vi "DSK.vi"() -> (0 "Total Money":i32, 1 "All TRansactions":string[][](table), 2 "Array 3":string[](array[string]), 3 "Current Transaction":string[][](table))   [LabVIEW 2023]
uses:
  <vilib>/Utility/file.llb/Read Delimited Spreadsheet (string).vi
panel:
  out "Waveform Chart":dbl(graph)
  in  "?":bool
  out "x .and. y?":bool
  out "Array 4":string[][](array[string])
  out "Array":string[][](array[string])
  out "Current Rows num":i32
  out "All Rows num":i32
  out "Array 2":string[](array[string])
  out "Transaction":string
  in  "Transaction Type":T1(ring)
  in  "file path":path
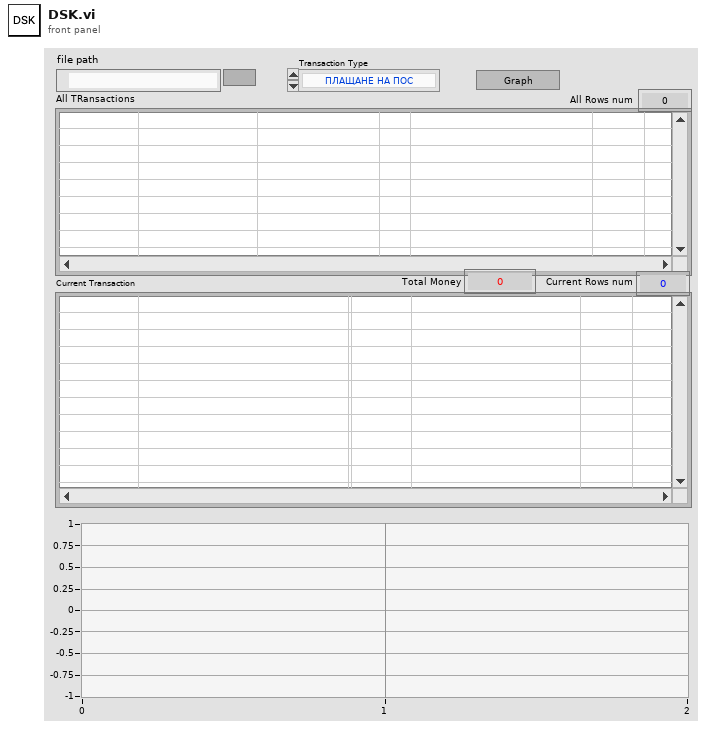
[diagram p1: front panel]
types:
  T1 = enum16{"ПЛАЩАНЕ НА ПОС", "СБКО", "ТЕГЛЕНЕ", "ЗАЕМ", "BREZOVO", "VIVACOM", "ЕЛЕКТРОХОЛД", "ЕВН", "ЗАПЛАТА", "АВАНС", "НЕТ", "ТРАНСФЕР"}
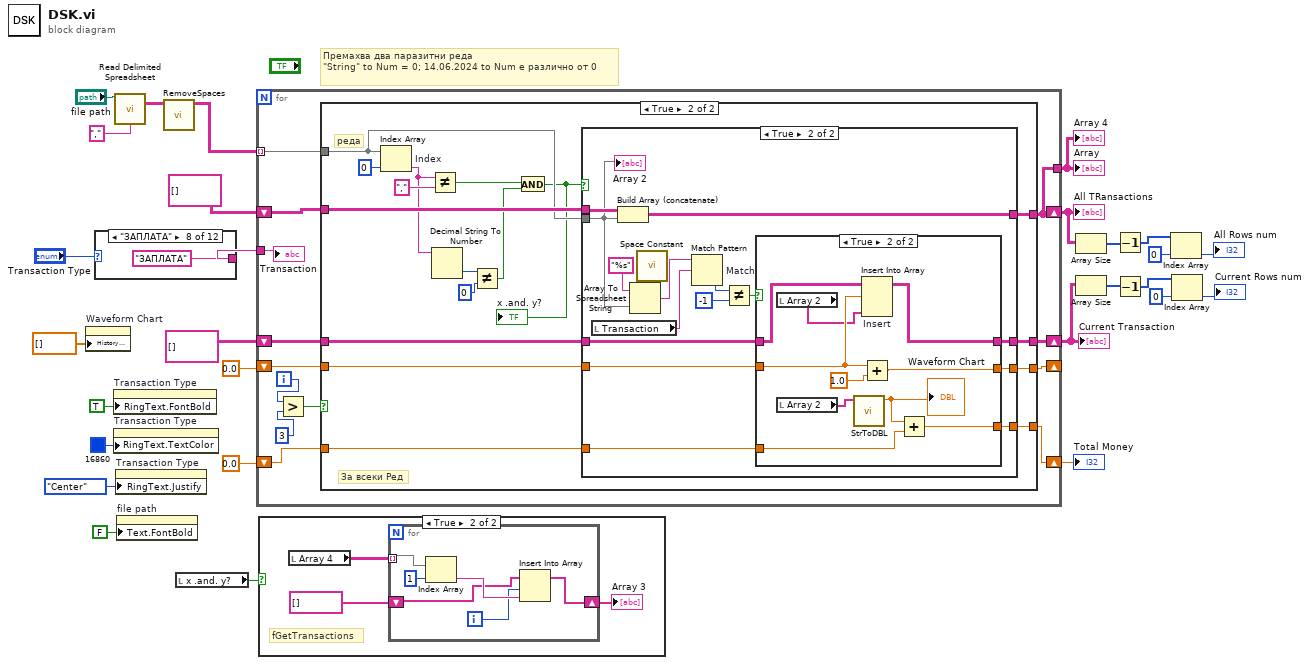
[diagram p0: block diagram]
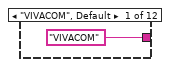
[diagram p3: hidden frame]
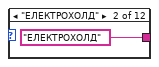
[diagram p4: hidden frame]
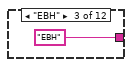
[diagram p5: hidden frame]
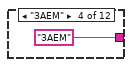
[diagram p6: hidden frame]
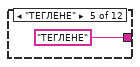
[diagram p7: hidden frame]
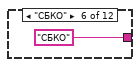
[diagram p8: hidden frame]
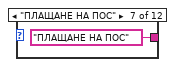
[diagram p9: hidden frame]
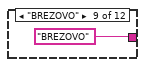
[diagram p10: hidden frame]
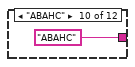
[diagram p11: hidden frame]
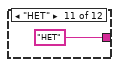
[diagram p12: hidden frame]
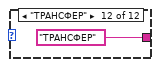
[diagram p13: hidden frame]
diagram:
  # "Премахва два паразитни реда\n\"String\" to Num = 0; 14.06.2024 to Num е различно от 0"
  n1 = property on="Waveform Chart" class="WFChart (strict)"("History Data"=dbl[] []) -> ()  [unwired: 2 in, 2 out]
  n2 = case shown="\"ЗАПЛАТА\"" "Transaction Type" {
    tunnel: ["VIVACOM" "ЕЛЕКТРОХОЛД" "ЕВН" "ЗАЕМ" "ТЕГЛЕНЕ" "СБКО" "ПЛАЩАНЕ НА ПОС" "ЗАПЛАТА" "BREZOVO" "АВАНС" "НЕТ" "ТРАНСФЕР"] -> w27
    frame "VIVACOM", Default {
    }
    frame "ЕЛЕКТРОХОЛД" {
    }
    frame "ЕВН" {
    }
    frame "ЗАЕМ" {
    }
    frame "ТЕГЛЕНЕ" {
    }
    frame "СБКО" {
    }
    frame "ПЛАЩАНЕ НА ПОС" {
    }
    frame "ЗАПЛАТА" {
    }
    frame "BREZOVO" {
    }
    frame "АВАНС" {
    }
    frame "НЕТ" {
    }
    frame "ТРАНСФЕР" {
    }
  }
  n3 = property on="Transaction Type" class="Enum (strict)"("RingText.FontBold"=TRUE ("Ring Text.Font:Bold")) -> ()  [unwired: 2 in, 2 out]
  n4 = property on="Transaction Type" class="Enum (strict)"("RingText.TextColor"=u32 16860 ("Ring Text.Text Colors:Text Color")) -> ()  [unwired: 2 in, 2 out]
  n5 = call-poly <vilib>:"Read Delimited Spreadsheet.vi"("file path (dialog if empty)"="file path", "delimiter (\\t)"="," ("delimiter (\\t)")) -> ("all rows"=w2:string[][])  [unwired: 8 in, 5 out]
  n6 = property on="Transaction Type" class="Enum (strict)"("RingText.Justify"=enum16{"Left", "Center", "Right"}."Center" ("Ring Text.Justification")) -> ()  [unwired: 2 in, 2 out]
  n7 = property on="file path" class="Path"("Text.FontBold"=FALSE ("Path Text.Font:Bold")) -> ()  [unwired: 2 in, 2 out]
  n8 = call "RemoveSpaces.vi"("all rows"=w2) -> ("Array 2"=w3:string[][])  [unwired: 10 in]
  n9 = local read "x .and. y?"() -> (w4:bool)
  n10 = for {
    tunnel: w27 -> [w49]
    tunnel: w3 -> [w45] mode=indexing
    shift-right: [w41] -> w19
    shift-left: string[][] [] -> [w50]
    shift-right: [w44] -> w6
    shift-left: string[][] [] -> [w48]
    shift-right: [w47] -> _
    shift-left: 0.0 ("y") -> [w46]
    shift-right: [w43] -> w18
    shift-left: 0.0 ("y") -> [w42]
    tunnel: [w41] -> w7
    i -> [w53]
    n11 = Greater?(x=w53, y=3) -> (0:w51:bool)
    n12 = case shown="True" w51 {
      tunnel: w45 -> [_ w65]
      tunnel: [w57 w72] -> w41
      tunnel: w50 -> [w57 w71]
      tunnel: [w56 w64] -> w44
      tunnel: w48 -> [w56 w63]
      tunnel: [w55 w62] -> w47
      tunnel: w46 -> [w55 w61]
      tunnel: [w54 w60] -> w43
      tunnel: w42 -> [w54 w59]
      frame False {
      }
      frame True {
        # "реда"
        # "За всеки Ред"
        n13 = Index Array "Index"(array=w65, index=0) -> (element=w70:string)
        n14 = Not Equal?(x=w70, y=",") -> (x != y?=w67:bool)
        n15 = Decimal String To Number(string=w70) -> (number=w69:i32)  [unwired: 2 in, 1 out]
        n16 = Not Equal?(x=w69, y=0) -> (x != y?=w66:bool)
        n17 = And(x=w67, y=w66) -> (x .and. y?=w58:bool)
        "x .and. y?" <- w58
        n18 = case shown="True" w58 {
          tunnel: w65 -> [_ w79]
          tunnel: [w78 w80] -> w72
          tunnel: w71 -> [w78 w94]
          tunnel: [w77 w83] -> w64
          tunnel: w63 -> [w77 w86]
          tunnel: [w76 w85] -> w62
          tunnel: w61 -> [w76 w84]
          tunnel: [w75 w82] -> w60
          tunnel: w59 -> [w75 w81]
          frame False {
          }
          frame True {
            n19 = local read "Transaction"() -> (w90:string)
            n20 = Build Array (concatenate)(w94, w79) -> (w80:string[][])
            n21 = call <vilib>:"Space Constant.vi"() -> ("String"=w92:string)
            n22 = Array To Spreadsheet String(delimiter (Tab)=w92, array=w79, 3:"%s" ("format string")) -> (spreadsheet string=w91:string)
            n23 = Match Pattern "Match"(string=w91, regular expression=w90) -> (offset past match=w89:i32)  [unwired: 1 in, 3 out]
            n24 = Not Equal?(x=w89, y=-1) -> (x != y?=w87:bool)
            n25 = case shown="True" w87 {
              tunnel: [w97 w99] -> w83
              tunnel: w86 -> [w97 w107]
              tunnel: [w96 w105] -> w85
              tunnel: w84 -> [w96 w104]
              tunnel: [w95 w101] -> w82
              tunnel: w81 -> [w95 w100]
              frame False {
              }
              frame True {
                n26 = local read "Array 2"() -> (w103:string[])
                n27 = local read "Array 2"() -> (w102:string[])
                n28 = call "StrToDBL.vi"("Array 2"=w102) -> ("number"=w98:dbl)  [unwired: 9 in, 1 out]
                "Waveform Chart" <- w98
                n29 = Insert Into Array "Insert"(array=w107, index (row)=w104, new element=w103) -> (w99:string[][])  [unwired: 1 in]
                n30 = Add(x=w104, y=1.0) -> (x+y=w105:dbl)
                n31 = Add(x=w98, y=w100) -> (x+y=w101:dbl)
              }
            }
            "Array 2" <- w79
          }
        }
      }
    }
    "Transaction" <- w49
  }
  "Current Transaction" <- w6
  "All TRansactions" <- w19
  "Total Money" <- w18
  "Array" <- w7
  "Array 4" <- w7
  n32 = case shown="True" w4 {
    frame False {
    }
    frame True {
      # "fGetTransactions"
      n33 = local read "Array 4"() -> (w110:string[][])
      n34 = for {
        tunnel: w110 -> [w116] mode=indexing
        shift-right: [w112] -> w108
        shift-left: string[] [] -> [w113]
        i -> [w111]
        n35 = Index Array(array=w116, index=1) -> (element=w114:string)
        n36 = Insert Into Array(array=w113, index=w111, new element=w114) -> (w112:string[])
      }
      "Array 3" <- w108
    }
  }
  n37 = Array Size(array=w19) -> (size(s)=w14:i32[])
  n38 = Array Size(array=w6) -> (size(s)=w12:i32[])
  n39 = Decrement(x=w14) -> (x-1=w13:i32[])
  n40 = Decrement(x=w12) -> (x-1=w11:i32[])
  n41 = Index Array(array=w13, index=0) -> (element=→"All Rows num":i32)
  n42 = Index Array(array=w11, index=0) -> (element=→"Current Rows num":i32)
